vi "UpdataUIData.vi"(8 "数组":string[](array[string]), 11 "表格输入":refnum<vi>) -> ()   [LabVIEW 2017]
uses:
  <vilib>/Utility/miscctls.llb/LVRowAndColumnUnsignedTypeDef.ctl
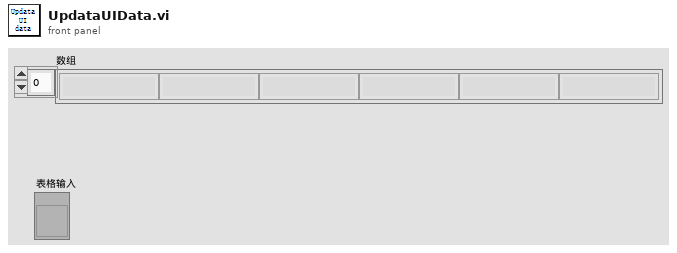
[diagram p1: front panel]
types:
  T1 = enum8{"Enabled", "Disabled", "Disabled and Grayed Out"}
  T2 = typedef "LVRowAndColumnUnsignedTypeDef.ctl" = cluster{"Row":u32, "Column":u32}
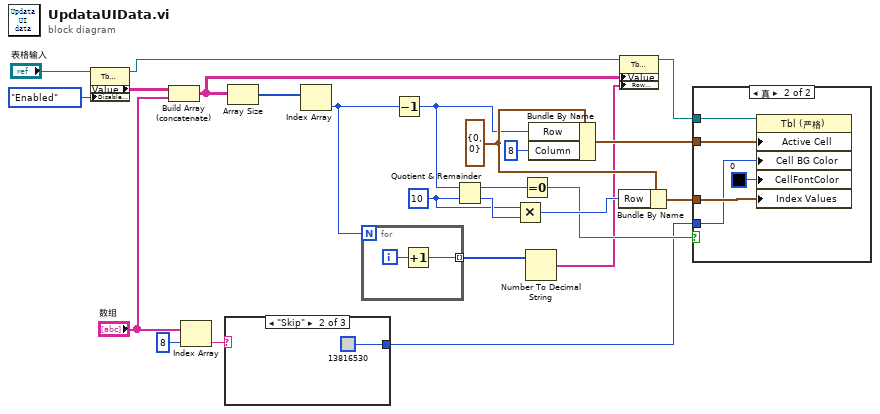
[diagram p0: block diagram]
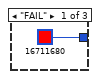
[diagram p2: hidden frame]
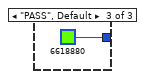
[diagram p3: hidden frame]
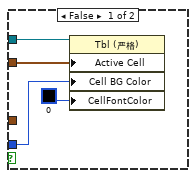
[diagram p4: hidden frame]
diagram:
  w16 = T2 {"Row"=0, "Column"=0} ("索引值")
  w17 = 10 ("y")
  n1 = property class="Tbl (严格)"(reference="表格输入", "DisabledEnum"=T1."Enabled" ("禁用")) -> (reference out=w15:refnum<vi>, "Value"=w23:string[][])  [unwired: 1 in, 1 out]
  n2 = Build Array (concatenate)(w23, "数组") -> (w22:string[][])
  n3 = Index Array(array="数组", index=8 ("索引")) -> (element=w10:string)
  n4 = case shown="\"Skip\"" w10 {
    tunnel: [u32 16711680 u32 13816530 u32 6618880] -> w11
    frame "FAIL" {
    }
    frame "Skip" {
    }
    frame "PASS", Default {
    }
  }
  n5 = Array Size(array=w22) -> (size(s)=w5:i32[])
  n6 = Index Array(array=w5) -> (element=w2:i32)  [unwired: 1 in]
  n7 = for {
    N: w2 -> [_]
    tunnel: [w28] -> w4 mode=indexing
    i -> [w29]
    n8 = Increment(x=w29) -> (x+1=w28:i32)
  }
  n9 = Decrement(x=w2) -> (x-1=w6:i32)
  n10 = Quotient & Remainder(x=w6, y=w17) -> (x-y*floor(x/y)=w20:i32, floor(x/y)=w19:i32)
  n11 = Multiply(x=w17, y=w19) -> (x*y=w18:i32)
  n12 = Equal To 0?(x=w20) -> (x = 0?=w13:bool)
  n13 = Number To Decimal String(number=w4) -> (decimal integer string=w3:string[])  [unwired: 1 in]
  n14 = Bundle By Name(cluster=w16, "Row"=w6, "Column"=8 ("X索引")) -> (w14:T2)
  n15 = Bundle By Name(cluster=w16, "Row"=w18) -> (w12:T2)
  n16 = property class="Tbl (严格)"(reference=w15, "Value"=w22, "Row Headers[]"=w3) -> (reference out=w7:refnum<vi>)  [unwired: 1 in, 1 out]
  n17 = case shown="真" w13 {
    tunnel: w7 -> [w31 w38]
    tunnel: w14 -> [w32 w37]
    tunnel: w12 -> [_ w36]
    tunnel: w11 -> [w33 w35]
    frame False {
      n18 = property class="Tbl (严格)"(reference=w31, "Active Cell"=w32, "Cell BG Color"=w33, "CellFontColor"=u32 0) -> ()  [unwired: 1 in, 2 out]
    }
    frame True {
      n19 = property class="Tbl (严格)"(reference=w38, "Active Cell"=w37, "Cell BG Color"=w35, "CellFontColor"=u32 0, "Index Values"=w36) -> ()  [unwired: 1 in, 2 out]
    }
  }
